vi "Deserialize Class.vi"(7 "Formatter":refnum<class "Formatter.lvclass">, 8 "error in":errorcluster, 10 "cfg path":path, 11 "Instrument In":refnum<class "Instrument.lvclass">) -> (0 "error out":errorcluster, 1 "text":string, 3 "Instrument Out":refnum<class "Instrument.lvclass">)   [LabVIEW 2012]
uses:
  <userlib>/Serialization/JSON Deserializer/JSON Deserializer.lvclass
  <userlib>/Serialization/Deserializer/Deserializer.lvclass
  <userlib>/Serialization/Formatter/Formatter.lvclass
  Instrument.lvclass
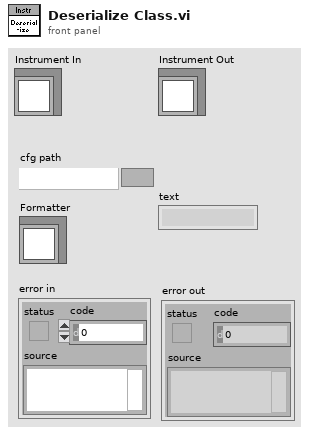
[diagram p1: front panel]
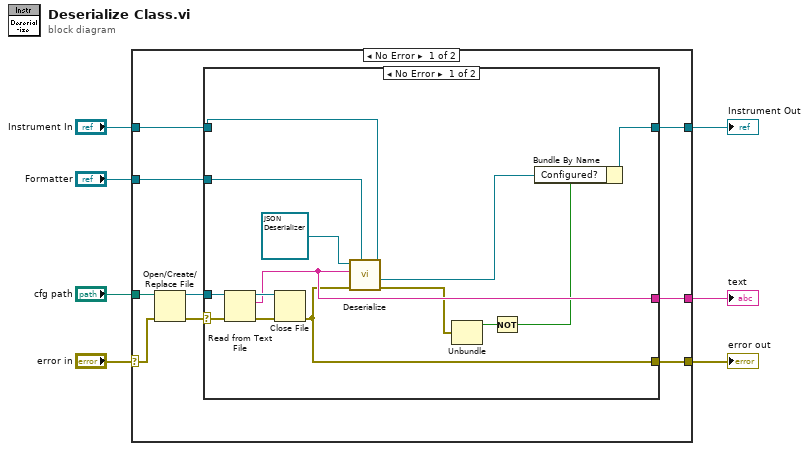
[diagram p0: block diagram]
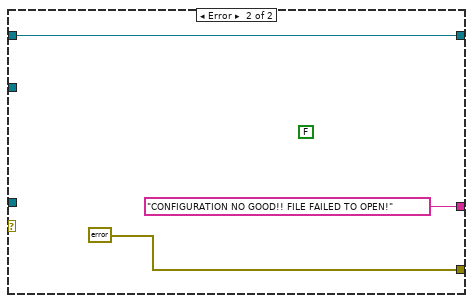
[diagram p2: hidden frame]
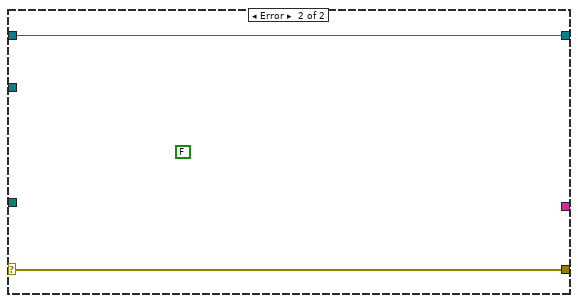
[diagram p3: hidden frame]
diagram:
  n1 = case shown="No Error" "error in" {
    selector: "error in" -> [w15 w35]
    tunnel: [w10 w35] -> w6
    tunnel: [w11 w34] -> w2
    tunnel: "Instrument In" -> [w12 w34]
    tunnel: "cfg path" -> [w16 _]
    tunnel: "Formatter" -> [w9 _]
    tunnel: [w8 _] -> w1
    frame No Error {
      n2 = Open/Create/Replace File(file path (use dialog)=w16, error in=w15) -> (refnum out=w13:refnum<file>, error out=w14:errorcluster)  [unwired: 4 in, 1 out]
      n3 = case shown="No Error" w14 {
        selector: w14 -> [w30 _]
        tunnel: w13 -> [w29 _]
        tunnel: w12 -> [w27 w33]
        tunnel: [w19 w33] -> w11
        tunnel: [w18 errorcluster {"status"=FALSE, "code"=0, "source"=""} ("error out")] -> w10
        tunnel: w9 -> [w23 _]
        tunnel: [w22 "CONFIGURATION NO GOOD!! FILE FAILED TO OPEN!"] -> w8
        frame No Error {
          n4 = Read from Text File(file (use dialog)=w29, error in=w30) -> (refnum out=w24:refnum<file>, text=w22:string, error out=w25:errorcluster)  [unwired: 2 in, 1 out]
          n5 = Close File(refnum=w24, error in=w25) -> (error out=w18:errorcluster)  [unwired: 1 out]
          n6 = call <userlib>:"Deserialize.vi"("Target Type (Serializable.lvclass)"=w27, "Formatter (defaults)"=w23, "error in (no error)"=w18, "String"=w22, "Deserializer"=refnum<class "JSON Deserializer.lvclass"> refnum ("JSON Deserializer.lvclass")) -> ("error out"=w17:errorcluster, "Serializable"=w21:refnum<class "Serializable.lvclass">)  [unwired: 4 in, 1 out]
          n7 = Unbundle(w17) -> ("status"=w26:bool)  [unwired: 2 out]
          n8 = Not(x=w26) -> (.not. x?=w20:bool)
          n9 = Bundle By Name(cluster=w21, "Configured?"=w20) -> (w19:refnum<class "Serializable.lvclass">)
        }
        frame Error {
          (unwired) FALSE
        }
      }
    }
    frame Error {
      (unwired) FALSE
    }
  }
  "error out" <- w6
  "text" <- w1
  "Instrument Out" <- w2
